vi "Test Worker Job Count Incremented.vi"(8 "error in (no error)":errorcluster, 11 "Cashier Test in":refnum<class "Cashier Test.lvclass">) -> (0 "error out":errorcluster, 3 "Cashier Test out":refnum<class "Cashier Test.lvclass">)   [LabVIEW 2020, in "Cashier Test.lvclass"]
uses:
  Cashier Test.lvclass
  C:/git/astemes-triarc-examples/source/Coffee Shop/Tests/Worker Test/Worker Test.lvclass
  C:/Program Files (x86)/National Instruments/LabVIEW 2020/vi.lib/Astemes/LUnit/Test Case.lvclass
  Support/Beverages/TypeDefs/Drink Type.ctl
  Support/Beverages/TypeDefs/Options.ctl
  Processes/People/Customers/Customer/Customer.lvclass
  Test Doubles/Stub Job Handler/Stub Job Handler.lvclass
  C:/git/astemes-triarc-examples/source/Coffee Shop/Processes/People/Process Job/Job Handler.lvclass
  <vilib>/Astemes/Triarc Framework/Process/Process.lvclass/Process.ctl
  <vilib>/Astemes/LUnit/Test Case.lvclass/Test Case.ctl
  664c3365-0d0e-4466-8c39-37d15edae733.vi
  <vilib>/Astemes/Triarc Framework/Support/Execution timer.vi
  <vilib>/Astemes/Triarc Framework/Process/Private/SubVIs/Wait for finish.vi
  <vilib>/Astemes/Triarc Framework/Process/Private/SubVIs/Set Lifecycle State.vi
  <vilib>/Astemes/Triarc Framework/Process/Protected/Messaging/Send Message.vi
  <vilib>/Astemes/LUnit/Core/LUnit Test Case/Private/Append Pass Result.vi
  <vilib>/Astemes/LUnit/Core/LUnit Test Case/Private/Append Fail Result.vi
  664c3365-0d0e-4466-8c39-37d15edae733.vi/9c5d11cd-9439-4240-a1ee-d9baace9c924.vi
  <vilib>/Astemes/Triarc Framework/Process/Private/SubVIs/Handle Debug Data.vi
  <vilib>/Astemes/LUnit/Core/LUnit Test Case/Private/Run In UI.vi
  <vilib>/Astemes/Triarc Framework/Logging/Log Debug.vi
  <vilib>/AdvancedString/1D String Array to Delimited String.vi
  <vilib>/Utility/High Resolution Relative Seconds.vi
  <vilib>/Utility/error.llb/Clear Errors.vi
  Processes/People/Workers/Worker/Worker.lvclass
  C:/Program Files (x86)/National Instruments/LabVIEW 2020/vi.lib/Astemes/Triarc Framework/Process/Process.lvclass
  <vilib>/Astemes/Triarc Framework/Support/Dequeue Broadcast Message.vi
  <vilib>/Astemes/Triarc Framework/Process/Public/Lifecycle/Get Lifecycle State.vi
  <vilib>/Utility/error.llb/Error Cluster From Error Code.vi
  <vilib>/Astemes/Triarc Framework/Process/Public/Read Name.vi
  <vilib>/Astemes/Triarc Framework/Callback/Callback.lvclass
  <vilib>/Astemes/Triarc Framework/Process/Process.lvclass
  Worker Test/Worker Test.lvclass
  Support/Order/Order.lvclass
  Support/Beverages/Beverage/Beverage.lvclass
  <vilib>/Astemes/Triarc Framework/Support/Broadcast Event Dequeuers.lvlib
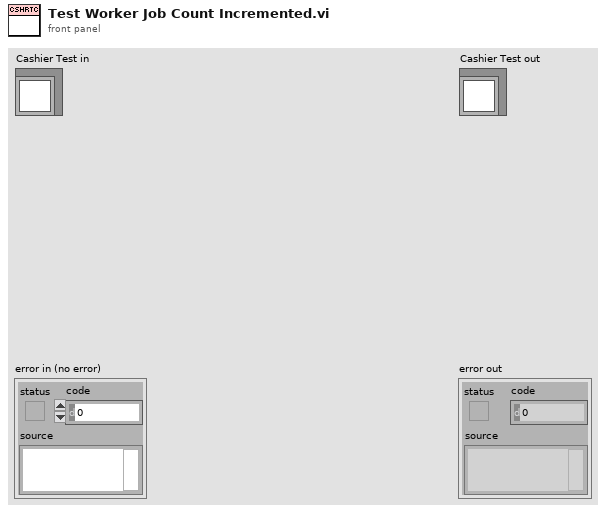
[diagram p1: front panel]
types:
  T1 = typedef "Beverage.lvclass/Drink Type.ctl" = enum16{"Dark Roast", "Decaf", "Espresso", "House Blend"}
  T2 = typedef "Beverage.lvclass/Options.ctl" = enum16{"<None>", "Milk", "Mocha", "Soy", "Whip"}
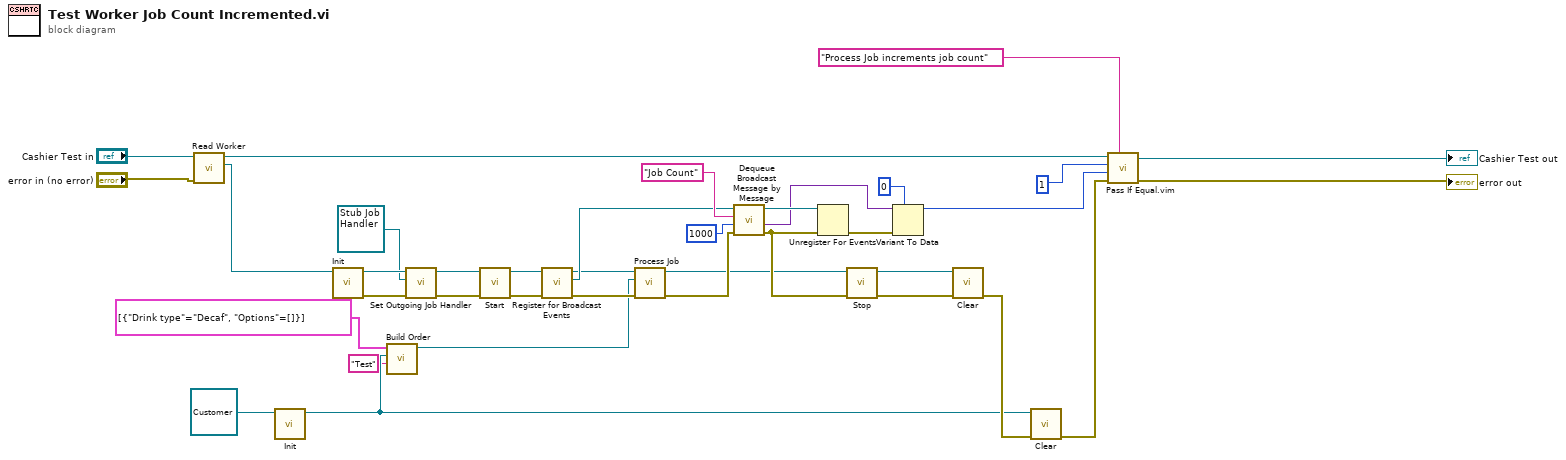
[diagram p0: block diagram]
diagram:
  n1 = call "Read Worker.vi"("error in (no error)"="error in (no error)", "Worker Test in"="Cashier Test in") -> ("Worker"=w13:refnum<class "Worker.lvclass">, "Worker Test out"=w12:refnum<class "Cashier Test.lvclass">)  [unwired: 7 in, 1 out]
  n2 = call-dynamic "Init.vi"("View In"=refnum<class "Customer.lvclass"> refnum ("Customer.lvclass")) -> ("View Out"=w7:refnum<class "Customer.lvclass">)  [unwired: 9 in, 1 out]
  n3 = call-dynamic "Init.vi"("View In"=w13) -> ("error out"=w14:errorcluster, "View Out"=w4:refnum<class "Worker.lvclass">)  [unwired: 9 in]
  n4 = call "Build Order.vi"("Customer Name"="Test", "Customer"=w7, "Order"=cluster{"Drink type":T1, "Options":T2[]}[] [{"Drink type"=enum."Decaf", "Options"=[]}]) -> ("Order Out"=w6:refnum<class "Order.lvclass">)  [unwired: 7 in, 1 out]
  n5 = call "Set Outgoing Job Handler.vi"("error in (no error)"=w14, "Work Dispatcher"=refnum<class "Stub Job Handler.lvclass"> refnum ("Stub Job Processor.lvclass"), "Worker In"=w4) -> ("error out"=w5:errorcluster, "Worker Out"=w3:refnum<class "Worker.lvclass">)  [unwired: 7 in]
  n6 = call <vilib>:"Start.vi"("error in (no error)"=w5, "Process In"=w3) -> ("error out"=w17:errorcluster, "Process Out"=w20:refnum<class "Worker.lvclass">)  [unwired: 7 in, 1 out]
  n7 = call <vilib>:"Register for Broadcast Events.vi"("error in (no error)"=w17, "Process In"=w20) -> ("error out"=w19:errorcluster, "Event Registration Refnum Out"=w24:refnum<event-registration>, "Process Out"=w21:refnum<class "Worker.lvclass">)  [unwired: 7 in]
  n8 = call-dynamic "Process Job.vi"("error in (no error)"=w19, "Job"=w6, "Worker In"=w21) -> ("error out"=w23:errorcluster, "Worker Out"=w22:refnum<class "Worker.lvclass">)  [unwired: 7 in]
  n9 = call <vilib>:"Dequeue Broadcast Message by Message.vi"("error in (no error)"=w23, "Timeout (-1)"=1000, "Message"="Job Count", "Event Registration Refnum"=w24) -> ("error out"=w30:errorcluster, "Message Data"=w27:variant, "Event Registration Refnum Out"=w33:refnum<event-registration>)  [unwired: 3 in, 2 out]
  n10 = Unregister For Events(event registration refnum=w33, error in=w30) -> (error out=w32:errorcluster)
  n11 = call <vilib>:"Stop.vi"("error in (no error)"=w30, "Process In"=w22) -> ("error out"=w16:errorcluster, "Process Out"=w15:refnum<class "Worker.lvclass">)  [unwired: 7 in, 1 out]
  n12 = Variant To Data(error in=w32, type=u32 0 ("code"), Variant=w27) -> (data=w29:u32)  [unwired: 1 out]
  n13 = call-dynamic "Clear.vi"("error in (no error)"=w16, "View In"=w15) -> ("error out"=w9:errorcluster)  [unwired: 9 in]
  n14 = call-dynamic "Clear.vi"("error in (no error)"=w9, "View In"=w7) -> ("error out"=w8:errorcluster)  [unwired: 9 in]
  n15 = call "Pass If Equal.vim"("Description"="Process Job increments job count", "error in (no error)"=w8, "Actual"=w29, "Expected"=u32 1 ("code"), "LUnit Test Case In"=w12) -> ("error out"=→"error out":errorcluster, "LUnit Test Case Out"=→"Cashier Test out":refnum<class "Cashier Test.lvclass">)  [unwired: 5 in]
